vi "OperationsCalc.vi"(10 "Fs":dbl format="%#_13g", 11 "RawData":dbl[][](array[numeric])) -> (2 "No Data?":bool, 3 "PropGraph":T1={"Raw Data"=[[0.0], [0.0234375], [0.9609375]], "Poperties"={"RMS values"=[], "Max"=[], "Min"=[], "A(8)"=[], "t"=0.0, "A(8) Axis"=0.0, "Aw"=[], "Ak 30min"=0.0, "Ak_axis"=0, "Spec"=[]}, "Power Spectrum / PSD"=[]})   [LabVIEW 2019]
uses:
  Communication/TypeDef/#TypeDef_PropGraph.ctl
  Communication/TypeDef/#TypeDef_PropertiesToSave.ctl
  Communication/TypeDef/#TypeDef_SetGet.ctl
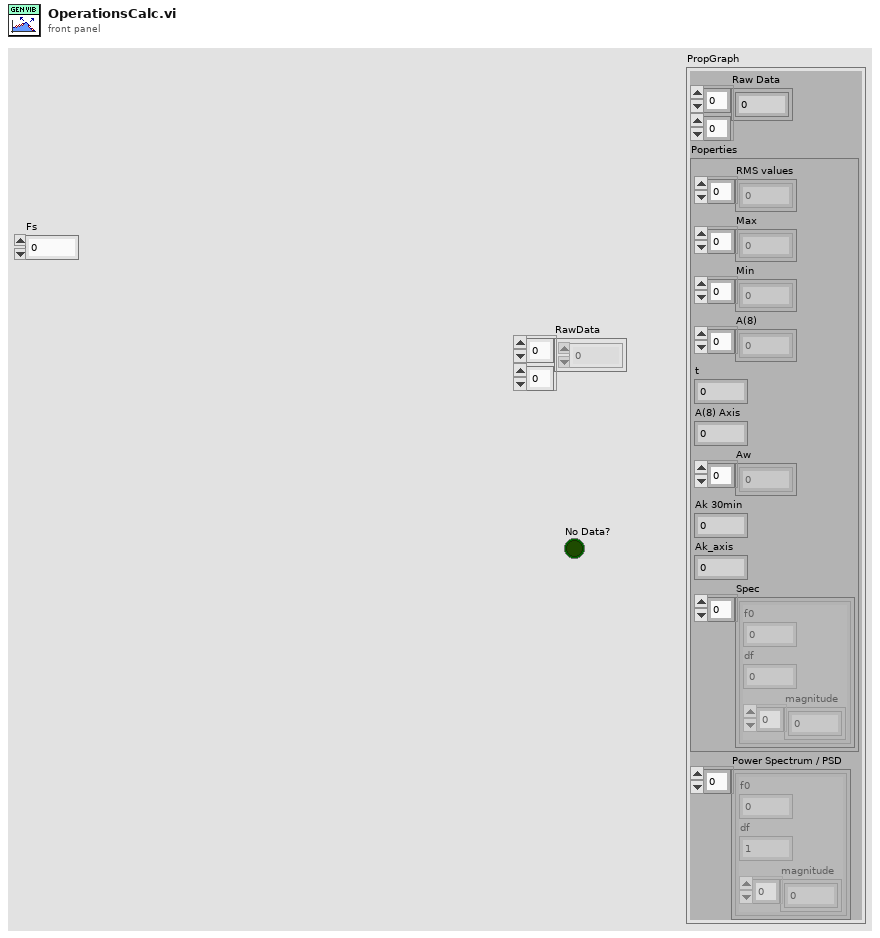
[diagram p1: front panel]
types:
  T1 = typedef "#TypeDef_PropGraph.ctl" = cluster{"Raw Data":dbl[][], "Poperties":T2, "Power Spectrum / PSD":cluster{"f0":dbl, "df":dbl, "magnitude":dbl[]}[]}
  T2 = typedef "#TypeDef_PropertiesToSave.ctl" = cluster{"RMS values":dbl[], "Max":dbl[], "Min":dbl[], "A(8)":dbl[], "t":dbl, "A(8) Axis":dbl, "Aw":dbl[], "Ak 30min":dbl, "Ak_axis":i32, "Spec":cluster{"f0":dbl, "df":dbl, "magnitude":dbl[]}[]}
  T3 = typedef "#TypeDef_SetGet.ctl" = enum16{"Set", "Get"}
  T4 = typedef "#TypeDef_MomentValues.ctl" = cluster{"Max":dbl[], "Min":dbl[], "RMS":dbl[], "Init?":bool}
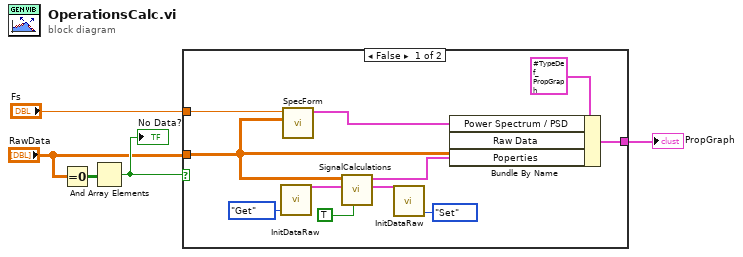
[diagram p0: block diagram]
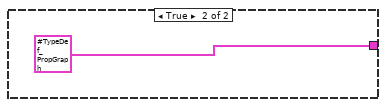
[diagram p2: hidden frame]
diagram:
  n1 = Equal To 0?(x="RawData") -> (x = 0?=w2:bool[][])
  n2 = And Array Elements(Boolean array=w2) -> (logical AND=w5:bool)
  "No Data?" <- w5
  n3 = case shown="False" w5 {
    tunnel: [w13 T1 {"Raw Data"=[[0.0], [0.0234375], [0.9609375]], "Poperties"={"RMS values"=[], "Max"=[], "Min"=[], "A(8)"=[], "t"=0.0, "A(8) Axis"=0.0, "Aw"=[], "Ak 30min"=0.0, "Ak_axis"=0, "Spec"=[]}, "Power Spectrum / PSD"=[]} ("PropGraph")] -> w4
    tunnel: "RawData" -> [w7 _]
    tunnel: "Fs" -> [w8 _]
    frame False {
      n4 = call "InitDataRaw.vi"("Get/Set"=#TypeDef_SetGet."Get") -> ("MomentValues Out"=w11:T4)  [unwired: 10 in]
      n5 = call "SpecForm.vi"("Data"=w7, "Fs"=w8) -> ("Power Spectrum / PSD"=w6:cluster{"f0":dbl, "df":dbl, "magnitude":dbl[]}[])  [unwired: 9 in]
      n6 = call "SignalCalculations.vi"("Ref?"=TRUE, "MomentValues in"=w11, "All Data"=w7) -> ("MomentValues Out"=w10:T4, "Poperties"=w12:T2)  [unwired: 7 in]
      n7 = call "InitDataRaw.vi"("Get/Set"=#TypeDef_SetGet."Set", "MomentValues in"=w10) -> ()  [unwired: 9 in, 1 out]
      n8 = Bundle By Name(cluster=T1 {"Raw Data"=[[0.0], [0.0234375], [0.9609375]], "Poperties"={"RMS values"=[], "Max"=[], "Min"=[], "A(8)"=[], "t"=0.0, "A(8) Axis"=0.0, "Aw"=[], "Ak 30min"=0.0, "Ak_axis"=0, "Spec"=[]}, "Power Spectrum / PSD"=[]} ("PropGraph"), "Power Spectrum / PSD"=w6, "Raw Data"=w7, "Poperties"=w12) -> (w13:T1)
    }
    frame True {
    }
  }
  "PropGraph" <- w4
